vi "실습 9-2.vi"() -> ()   [LabVIEW 2014]
panel:
  out "에러 출력":errorcluster
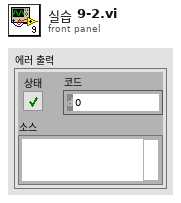
[diagram p1: front panel]
types:
  T1 = enum16{"open", "replace", "create", "open or create", "replace or create", "replace or create with confirmation"}
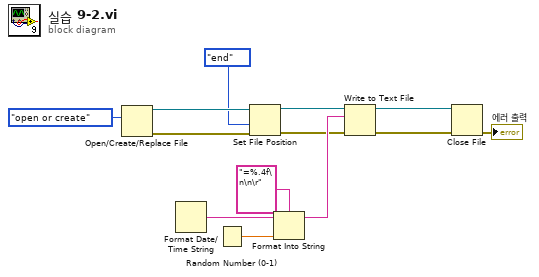
[diagram p0: block diagram]
diagram:
  n1 = Open/Create/Replace File(operation (0:open)=T1."open or create" ("동작(0:open)")) -> (refnum out=w4:refnum<file>, error out=w5:errorcluster)  [unwired: 5 in, 1 out]
  n2 = Format Date/Time String() -> (date/time string=w9:string)  [unwired: 3 in]
  n3 = Random Number (0-1)() -> (number: 0 to 1=w10:dbl)
  n4 = Set File Position(refnum=w4, from (0:start)=enum16{"start", "end", "current"}."end" ("시작(0:시작)"), error in=w5) -> (refnum out=w2:refnum<file>, error out=w1:errorcluster)  [unwired: 1 in]
  n5 = Format Into String(format string="=%.4f\n\n\r" ("포맷 문자열"), initial string=w9, w10) -> (resulting string=w7:string)  [unwired: 1 in, 1 out]
  n6 = Write to Text File(file (use dialog)=w2, text=w7, error in=w1) -> (refnum out=w13:refnum<file>, error out=w12:errorcluster)  [unwired: 1 in, 1 out]
  n7 = Close File(refnum=w13, error in=w12) -> (error out=→"에러 출력":errorcluster)  [unwired: 1 out]
